vi "httpsend.vi"(8 "error in (no error)":errorcluster caption="错误输入（无错误）", 11 "HTTP发送 输入":refnum<class "HTTP发送.lvclass">) -> (0 "error out":errorcluster caption="错误输出", 3 "HTTP发送 输出":refnum<class "HTTP发送.lvclass">)   [LabVIEW 2022 SP3, in "工况数据上传.lvlib" / "HTTP发送.lvclass"]
uses:
  C:/Program Files (x86)/National Instruments/LabVIEW 2022/vi.lib/ActorFramework/Actor/Actor.lvclass
  <vilib>/ActorFramework/Actor/Actor.lvclass/Actor.ctl
  <vilib>/ActorFramework/Message Enqueuer/Message Enqueuer.lvclass/Message Enqueuer.ctl
  <vilib>/ActorFramework/Message Enqueuer/Init from Existing Queue.vi
  <vilib>/ActorFramework/Message Enqueuer/Enqueue.vi
  C:/Program Files (x86)/National Instruments/LabVIEW 2022/vi.lib/ActorFramework/Message/Message.lvclass
  <vilib>/httpClient/POSTBuffer.vi
  <vilib>/ActorFramework/Message Priority Queue/Priority Enqueue.vi
  <vilib>/ActorFramework/Message Enqueuer/Message Enqueuer.lvclass
  <vilib>/httpClient/LabVIEWHTTPClient.lvlib
  <vilib>/ActorFramework/Actor/Actor.lvclass
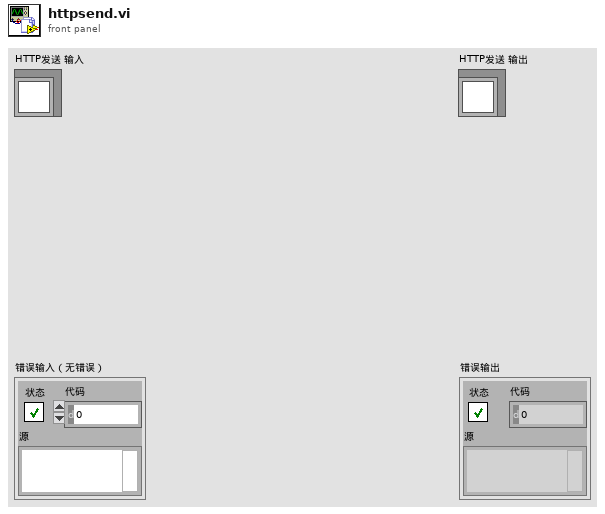
[diagram p1: front panel]
types:
  T1 = cluster{"url":string, "loginTokenRequest":cluster{"clientId":string, "clientSecret":string, "grantType":string, "password":string, "scope":string, "userName":string, "userType":string}, "自动获取MN":bool}
  T2 = cluster{"code":string, "message":string, "timestamp":u64, "data":cluster{"bearerType":string, "oauth2Type":string, "accessToken":string, "tokenType":string, "expiresIn":u64, "refreshToken":string, "scope":string[], "tokenDetail":cluster{"dataSource":string, "username":string, "userId":string, "userType":string, "enabled":bool, "accountNonExpired":bool, "credentialsNonExpired":bool, "accountNonLocked":bool}}, "success":bool}
  T3 = typedef "LabVIEWHTTPClient.lvlib/ClientHandle.ctl" = refnum<k1>
  T4 = typedef "工况数据.ctl" = cluster{"time":string, "data":cluster{"ups":cluster{"ups":cluster{"input_voltage":ext, "input_frequency":ext, "output_voltage":ext, "output_current":ext, "output_frequency":ext, "output_active_power":ext, "output_apparent_power":ext, "load_rate":ext, "cabinet_temperature":ext, "battery_voltage":ext, "remaining_battery_capacity":ext, "power_on_status":string, "power_supply_mode":string, "fault":bool, "battery_low_voltage":bool, "mains_supply_abnormality":bool}, "启用":bool}, "air_conditioner":cluster{"air_conditioner":cluster{"cabinet_temperature":ext, "air_supply_temperature":ext, "voltage":ext, "current":ext, "compressor_status":string, "Internal_fan_status":string, "external_fan_status":string, "heating_state":string, "refrigeration_state":bool, "high_temperature_alarm":bool, "low_temperature_alarm":bool, "heater_fault":bool, "temperature_sensor_fault":bool, "high_voltage_alarm":bool, "low_voltage_alarm":bool, "refrigeration_start_point":ext, "refrigeration_sensitive_point":ext, "heating_start_point":ext, "heating_sensitive_point":ext, "high_temperature_alarm_point":ext, "low_temperature_alarm_point":ext}, "启用":bool}, "smoke_sensor":cluster{"smoke_sensor":cluster{"trigger_alarm":bool}, "启用":bool}, "water_immersion_sensor":cluster{"water_immersion_sensor":cluster{"trigger_alarm":bool}, "启用":bool}, "temperature_and_humidity_sensor":cluster{"temperature_and_humidity_sensor":cluster{"current_temperature":ext, "current_humidity":ext, "room_temperature_alarm":bool, "humidity_alarm":bool}, "启用":bool}, "gps":cluster{"gps":cluster{"current_longitude":ext, "current_latitude":ext, "launch_longitude":ext, "launch_latitude":ext, "shift_alarm":bool}, "启用":bool}, "solar_controller":cluster{"solar_controller":cluster{"array_voltage":ext, "array_current":ext, "generating_power":ext, "battery_voltage":dbl, "battery_current":ext, "ceiling_voltage":ext, "minimum_voltage":ext, "battery_temperature":ext, "remaining_battery_capacity":ext, "load_voltage":ext, "load_current":ext, "load_power":ext, "equipment_temperature":ext, "accumulated_electricity_consumption_of_the_day":ext, "accumulated_electricity_consumption_of_the_current_month":ext, "accumulated_electricity_consumption_in_the_current_year":ext, "total_accumulated_power_consumption":ext, "accumulated_charging_capacity_of_the_day":ext, "accumulated_charging_amount_of_the_current_month":ext, "accumulated_charging_capacity_of_the_current_year":ext, "total_cumulative_charge":ext}, "启用":bool}, "solar_controller_2":cluster{"solar_controller_2":cluster{"array_voltage":ext, "array_current":ext, "generating_power":ext, "battery_voltage":dbl, "battery_current":ext, "ceiling_voltage":ext, "minimum_voltage":ext, "battery_temperature":ext, "remaining_battery_capacity":ext, "load_voltage":ext, "load_current":ext, "load_power":ext, "equipment_temperature":ext, "accumulated_electricity_consumption_of_the_day":ext, "accumulated_electricity_consumption_of_the_current_month":ext, "accumulated_electricity_consumption_in_the_current_year":ext, "total_accumulated_power_consumption":ext, "accumulated_charging_capacity_of_the_day":ext, "accumulated_charging_amount_of_the_current_month":ext, "accumulated_charging_capacity_of_the_current_year":ext, "total_cumulative_charge":ext}, "启用":bool}, "NH3":cluster{"NH3":cluster{"F0":ext, "F1":ext, "syringe_temperature":ext, "alarm_step":dbl, "X0":ext}, "启用":bool}, "TP":cluster{"TP":cluster{"F0":ext, "F1":ext, "F2":ext, "F3":ext, "digestion_temperature":ext, "constant_temperature":ext, "syringe_temperature":ext, "alarm_step":dbl, "X0":ext}, "启用":bool}, "TN":cluster{"TN":cluster{"F0":ext, "F1":ext, "F2":ext, "F3":ext, "F4":ext, "F5":ext, "F6":ext, "F7":ext, "digestion_temperature":ext, "constant_temperature":ext, "syringe_temperature":ext, "alarm_step":dbl, "X0":ext}, "启用":bool}, "CODMn":cluster{"CODMn":cluster{"temperature_curve":ext[], "titration_curve":ext[], "F0":ext, "F1":ext, "F2":ext, "F3":ext, "F4":ext, "F5":ext, "A":ext, "B":ext, "K":ext}, "启用":bool}, "CODCr":cluster{"CODCr":cluster{"temperature_curve":ext[], "F0":ext, "F1":ext, "reagent_sensor":ext}, "启用":bool}}}
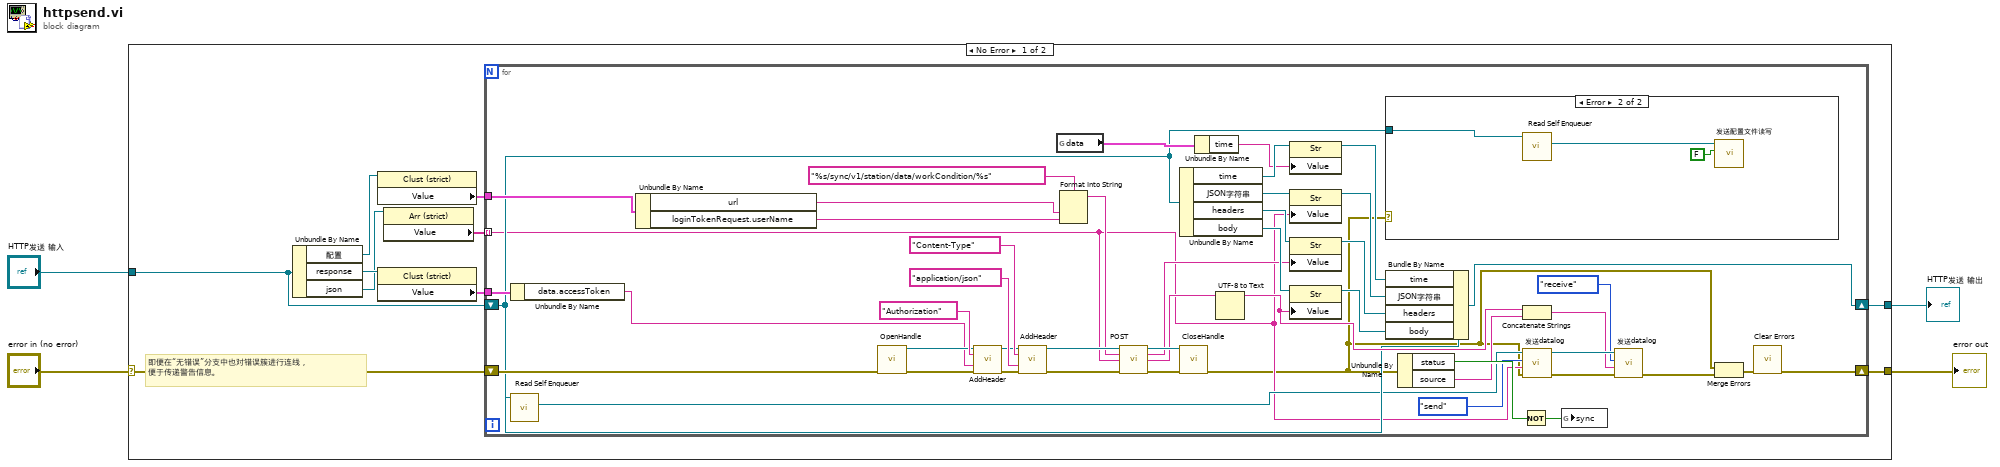
[diagram p0: block diagram]
diagram:
  n1 = case shown="No Error" "error in (no error)" {
    selector: "error in (no error)" -> [w10 w67]
    tunnel: [w5 w67] -> w3
    tunnel: [w6 w66] -> w1
    tunnel: "HTTP发送 输入" -> [w7 w66]
    frame No Error {
      # "即便在“无错误”分支中也对错误簇进行连线，\n便于传递警告信息。"
      n2 = Unbundle By Name(w7) -> ("配置"=w14:refnum<vi>, "response"=w13:refnum<vi>, "json"=w12:refnum<vi>)
      n3 = property class="Clust (strict)"(reference=w14) -> ("Value"=w11:T1)  [unwired: 1 in, 2 out]
      n4 = property class="Clust (strict)"(reference=w13) -> ("Value"=w8:T2)  [unwired: 1 in, 2 out]
      n5 = property class="Arr (strict)"(reference=w12) -> ("Value"=w9:string[])  [unwired: 1 in, 2 out]
      n6 = for {
        shift-right: [w36] -> w6
        shift-left: w7 -> [w24]
        shift-right: [w37] -> w5
        shift-left: w10 -> [w39]
        tunnel: w9 -> [w21] mode=indexing
        tunnel: w11 -> [w42]
        tunnel: w8 -> [w40]
        n7 = Unbundle By Name(w40) -> ("data.accessToken"=w50:string)
        n8 = call <vilib>:"Read Self Enqueuer.vi"("Actor"=w24) -> ("Self Enqueuer"=w23:refnum<class "Message Enqueuer.lvclass">)  [unwired: 10 in]
        n9 = Unbundle By Name(w42) -> ("url"=w48:string, "loginTokenRequest.userName"=w47:string)
        n10 = call <vilib>:"OpenHandle.vi"("error in (no error)"=w39) -> ("client handle out"=w53:T3, "error out"=w52:errorcluster)  [unwired: 13 in]
        n11 = call <vilib>:"AddHeader.vi"("client handle"=w53, "header"="Authorization", "value"=w50, "error in (no error)"=w52) -> ("client handle out"=w54:T3, "error out"=w51:errorcluster)  [unwired: 10 in]
        n12 = call <vilib>:"AddHeader.vi"("client handle"=w54, "header"="Content-Type", "value"="application/json", "error in (no error)"=w51) -> ("client handle out"=w57:T3, "error out"=w56:errorcluster)  [unwired: 10 in]
        n13 = global read "工况数据接口全局.vi" "data"() -> (w41:T4)
        n14 = Format Into String(format string="%s/sync/v1/station/data/workCondition/%s" ("url"), w48, w47) -> (resulting string=w46:string)  [unwired: 2 in, 1 out]
        n15 = call-poly <vilib>:"POST.vi"("client handle"=w57, "url"=w46, "buffer"=w21, "error in (no error)"=w56) -> ("client handle out"=w60:T3, "headers"=w26:string, "body"=w58:string, "error out"=w59:errorcluster)  [unwired: 8 in]
        n16 = Unbundle By Name(w24) -> ("time"=w35:refnum<vi>, "JSON字符串"=w34:refnum<vi>, "headers"=w33:refnum<vi>, "body"=w32:refnum<vi>)
        n17 = call <vilib>:"CloseHandle.vi"("client handle"=w60, "error in (no error)"=w59) -> ("error out"=w20:errorcluster)  [unwired: 13 in]
        n18 = Unbundle By Name(w41) -> ("time"=w25:string)
        n19 = UTF-8 to Text(11:w58) -> (3:w27:string)  [unwired: 2 in, 1 out]
        n20 = property class="Str"(reference=w35, "Value"=w25) -> (reference out=w31:refnum<vi>)  [unwired: 1 in, 1 out]
        n21 = property class="Str"(reference=w34, "Value"=w21) -> (reference out=w30:refnum<vi>)  [unwired: 1 in, 1 out]
        n22 = property class="Str"(reference=w33, "Value"=w26) -> (reference out=w29:refnum<vi>)  [unwired: 1 in, 1 out]
        n23 = property class="Str"(reference=w32, "Value"=w27) -> (reference out=w28:refnum<vi>)  [unwired: 1 in, 1 out]
        n24 = case shown="Error" w20 {
          tunnel: w24 -> [_ w65]
          frame No Error {
          }
          frame Error {
            n25 = call <vilib>:"Read Self Enqueuer.vi"("Actor"=w65) -> ("Self Enqueuer"=w64:refnum<class "Message Enqueuer.lvclass">)  [unwired: 10 in]
            n26 = call "发送配置文件读写.vi"("write?"=FALSE, "Message Enqueuer"=w64) -> ()  [unwired: 8 in, 2 out]
          }
        }
        n27 = Bundle By Name(cluster=w24, "time"=w31, "JSON字符串"=w30, "headers"=w29, "body"=w28) -> (w36:refnum<class "HTTP发送.lvclass">)
        n28 = Unbundle By Name(w20) -> ("status"=w45:bool, "source"=w43:string)
        n29 = Not(x=w45) -> (.not. x?=w44:bool)
        n30 = Concatenate Strings(w27, w43) -> (w17:string)
        n31 = call "发送datalog.vi"("error in (no error)"=w20, "data"=w21, "send/receive"=enum16{"send", "receive"}."send", "Message Enqueuer"=w23) -> ("error out"=w18:errorcluster, "Message Enqueuer out"=w19:refnum<class "Message Enqueuer.lvclass">)  [unwired: 6 in]
        n32 = global write "工况数据接口全局.vi" "sync"(w44) -> ()
        n33 = call "发送datalog.vi"("error in (no error)"=w18, "data"=w17, "send/receive"=enum16{"send", "receive"}."receive", "Message Enqueuer"=w19) -> ("error out"=w15:errorcluster)  [unwired: 6 in, 1 out]
        n34 = Merge Errors(w20, w15) -> (w38:errorcluster)
        n35 = call <vilib>:"Clear Errors.vi"("error in (no error)"=w38) -> ("error out"=w37:errorcluster)  [unwired: 5 in, 1 out]
      }
    }
    frame Error {
    }
  }
  "error out" <- w3
  "HTTP发送 输出" <- w1
